vi "Analyze Eyes.vi"(7 "Fixation radius":dbl=50.0, 10 "Input":variant, 11 "Data":T1) -> (2 "Fixated":bool)   [LabVIEW 2011]
uses:
  Z:/libraries/Labview/Core SubVIs/Controls/TYPE - Analog Data.ctl
  <vilib>/Waveform/WDTOps.llb/WDT Waveform Duration DBL.vi
  Z:/libraries/Labview/Core SubVIs/Core SubVIs.lvlib
panel:
  out "Horizontal":waveform(dbl)(graph)
  out "Vertical":waveform(dbl)(graph)
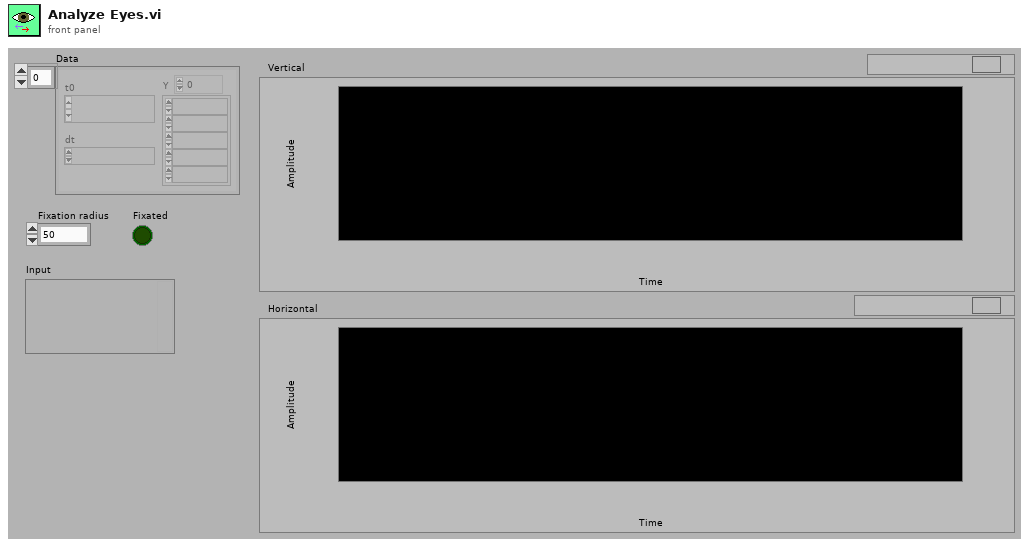
[diagram p1: front panel]
types:
  T1 = typedef "Core SubVIs.lvlib/TYPE - Analog Data.ctl" = waveform(dbl)[]
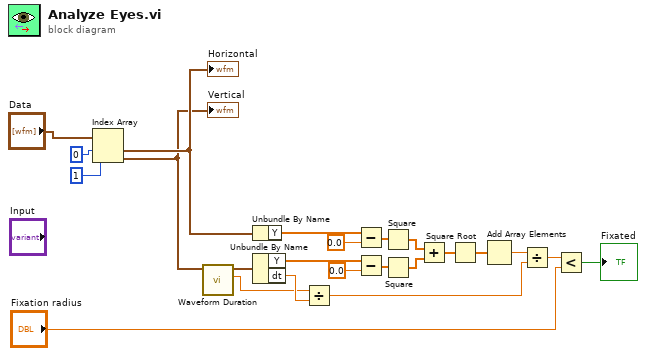
[diagram p0: block diagram]
diagram:
  n1 = Index Array(array="Data", index #1=0 ("index"), index #2=1 ("index")) -> (element #1=w3:waveform(dbl), element #2=w1:waveform(dbl))
  "Vertical" <- w1
  "Horizontal" <- w3
  n2 = call-poly <vilib>:"Waveform Duration.vi"("waveform in"=w1) -> ("duration"=w8:dbl, "waveform out"=w10:waveform(dbl))  [unwired: 8 in, 1 out]
  n3 = Unbundle By Name(w3) -> ("Y"=w2:dbl[])
  n4 = Unbundle By Name(w10) -> ("Y"=w14:dbl[], "dt"=w9:dbl)
  n5 = Divide(x=w8, y=w9) -> (x/y=w7:dbl)
  n6 = Subtract(x=w2, y=0.0 ("X")) -> (x-y=w19:dbl[])
  n7 = Subtract(x=w14, y=0.0 ("X")) -> (x-y=w17:dbl[])
  n8 = Square(x=w19) -> (x^2=w18:dbl[])
  n9 = Square(x=w17) -> (x^2=w15:dbl[])
  n10 = Add(x=w18, y=w15) -> (x+y=w13:dbl[])
  n11 = Square Root(x=w13) -> (sqrt(x)=w12:dbl[])
  n12 = Add Array Elements(numeric array=w12) -> (sum=w11:dbl)
  n13 = Divide(x=w11, y=w7) -> (x/y=w6:dbl)
  n14 = Less?(x=w6, y="Fixation radius") -> (x < y?=→"Fixated":bool)
